vi "flattenLengthToXML_Scalar.vi"(8 "error in (no error)":errorcluster, 9 "lengthUnitInXML":T1, 10 "lengthAgain":variant, 11 "length":dbl[unit]) -> (0 "error out":errorcluster, 3 "xmlString":string)   [LabVIEW 2016, in "UnitsAndXML.lvlib"]
uses:
  <userlib>/Common/UnitsAndXML/UnitsAndXML.lvlib
  <userlib>/Common/UnitsAndXML/FlattenItemWithUnitToXML/FlattenLengthToXML/LengthUnit.ctl
  <vilib>/Utility/VariantDataType/VariantType.lvlib
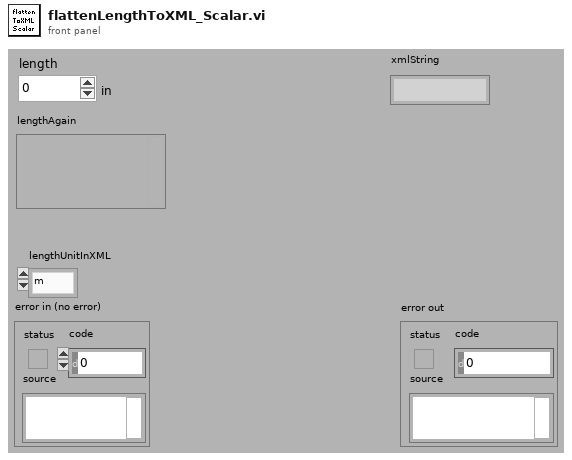
[diagram p1: front panel]
types:
  T1 = typedef "UnitsAndXML.lvlib/LengthUnit.ctl" = enum16{"m", "Angstrom", "AU", "chain", "cm", "cubit", "fathom", "fermi", "ft", "furlong", "hubble", "in", "ly", "mi", "mm", "rod", "um", "yd"}
  T2 = typedef "VariantType.lvlib/Type.ctl" = enum8{"Invalid Type", "Void", "I8", "I16", "I32", "I64", "U8", "U16", "U32", "U64", "Single Float", "Double Float", "Extended Float", "Single Complex", "Double Complex", "Extended Complex", "Enum U8", "Enum U16", "Enum U32", "Enum U64", "Single Float With Unit", "Double Float With Unit", "Extended Float With Unit", "Single Complex with Unit", "Double Complex with Unit", "Extended Complex with Unit", "Boolean", "String", "Path", "Picture", "Tag", "Array", "Cluster", "Variant", "LV Variant", "Waveform", "Timestamp", "Digital Waveform", "Digital Data", "ExpressData", "Refnum", "External Data", "VI", "Poly VI", "LabVIEW Class Instance", "Fixed Point"}
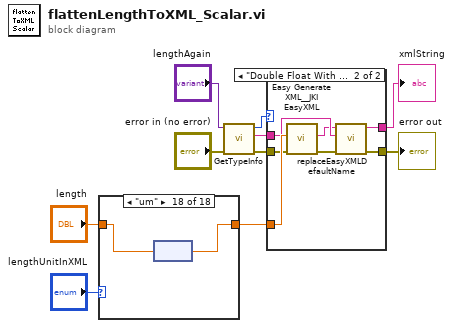
[diagram p0: block diagram]
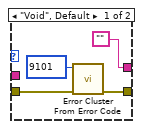
[diagram p2: hidden frame]
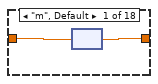
[diagram p3: hidden frame]
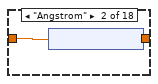
[diagram p4: hidden frame]
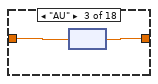
[diagram p5: hidden frame]
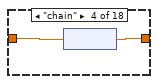
[diagram p6: hidden frame]
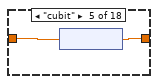
[diagram p7: hidden frame]
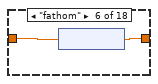
[diagram p8: hidden frame]
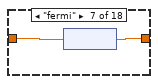
[diagram p9: hidden frame]
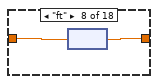
[diagram p10: hidden frame]
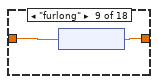
[diagram p11: hidden frame]
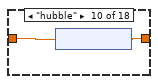
[diagram p12: hidden frame]
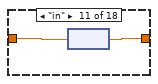
[diagram p13: hidden frame]
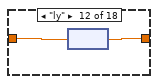
[diagram p14: hidden frame]
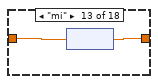
[diagram p15: hidden frame]
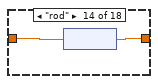
[diagram p16: hidden frame]
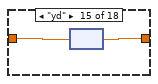
[diagram p17: hidden frame]
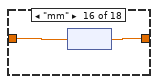
[diagram p18: hidden frame]
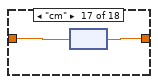
[diagram p19: hidden frame]
diagram:
  n1 = case shown="\"um\"" "lengthUnitInXML" {
    tunnel: "length" -> [w12 w14 w16 w18 w19 w22 w24 w26 w28 w30 w32 w34 w36 w38 w40 w42 w44 w46]
    tunnel: [w11 w13 w15 w17 w20 w21 w23 w25 w27 w29 w31 w33 w35 w37 w39 w41 w43 w45] -> w10
    frame "m", Default {
      n2 = node(w12) -> (w11:dbl)
    }
    frame "Angstrom" {
      n3 = node(w14) -> (w13:dbl)
    }
    frame "AU" {
      n4 = node(w16) -> (w15:dbl)
    }
    frame "chain" {
      n5 = node(w18) -> (w17:dbl)
    }
    frame "cubit" {
      n6 = node(w19) -> (w20:dbl)
    }
    frame "fathom" {
      n7 = node(w22) -> (w21:dbl)
    }
    frame "fermi" {
      n8 = node(w24) -> (w23:dbl)
    }
    frame "ft" {
      n9 = node(w26) -> (w25:dbl)
    }
    frame "furlong" {
      n10 = node(w28) -> (w27:dbl)
    }
    frame "hubble" {
      n11 = node(w30) -> (w29:dbl)
    }
    frame "in" {
      n12 = node(w32) -> (w31:dbl)
    }
    frame "ly" {
      n13 = node(w34) -> (w33:dbl)
    }
    frame "mi" {
      n14 = node(w36) -> (w35:dbl)
    }
    frame "rod" {
      n15 = node(w38) -> (w37:dbl)
    }
    frame "yd" {
      n16 = node(w40) -> (w39:dbl)
    }
    frame "mm" {
      n17 = node(w42) -> (w41:dbl)
    }
    frame "cm" {
      n18 = node(w44) -> (w43:dbl)
    }
    frame "um" {
      n19 = node(w46) -> (w45:dbl)
    }
  }
  n20 = call <vilib>:"GetTypeInfo.vi"("error in (no error)"="error in (no error)", "Variant"="lengthAgain") -> ("error out"=w2:errorcluster, "Name"=w1:string, "Type Enum"=w3:T2)  [unwired: 5 in, 2 out]
  n21 = case shown="\"Double Float With Unit\"" w3 {
    tunnel: w10 -> [_ w57]
    tunnel: ["" w56] -> w7
    tunnel: [w49 w55] -> w6
    tunnel: w2 -> [w47 w52]
    tunnel: w1 -> [_ w54]
    frame "Void", Default {
      n22 = call <vilib>:"Error Cluster From Error Code.vi"("error in (no error)"=w47, "error code (0)"=9101) -> ("error out"=w49:errorcluster)  [unwired: 7 in]
    }
    frame "Double Float With Unit" {
      n23 = call <vilib>:"Easy Generate XML__JKI EasyXML.vi"("error in (no error)"=w52, "LabVIEW Data"=w57) -> ("error out"=w51:errorcluster, "XML String"=w53:string)  [unwired: 8 in]
      n24 = call <userlib>:"replaceEasyXMLDefaultName.vi"("error in"=w51, "desiredName"=w54, "easyXMLStringWithDefaultNames"=w53) -> ("error out"=w55:errorcluster, "xmlString"=w56:string)  [unwired: 7 in]
    }
  }
  "xmlString" <- w7
  "error out" <- w6
